vi "writeRequest.vi"(5 "id":u16, 7 "cmd":string, 9 "data":string) -> (8 "readRequest":string)   [LabVIEW 2015, in "labOpenShowVar.lvlib"]
uses:
  labOpenShowVar.lvlib
panel:
  out "输出":u8[](array[numeric]) format="%02d"
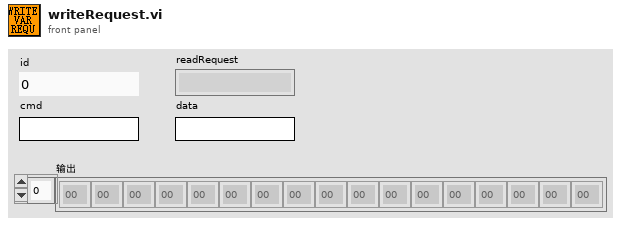
[diagram p1: front panel]
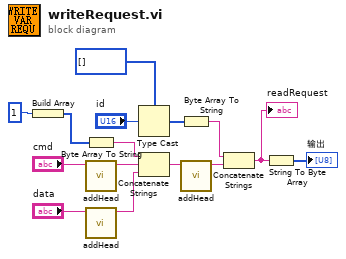
[diagram p0: block diagram]
diagram:
  n1 = Build Array(u8 1) -> (w9:u8[])
  n2 = Byte Array To String(unsigned byte array=w9) -> (string=w12:string)
  n3 = call "addHead.vi"("cmd"="cmd") -> ("添加后"=w13:string)  [unwired: 10 in]
  n4 = call "addHead.vi"("cmd"="data") -> ("添加后"=w1:string)  [unwired: 10 in]
  n5 = Type Cast(type=u8[] [], x="id") -> (*(type *) &x=w3:u8[])
  n6 = Concatenate Strings(w12, w13, w1) -> (w11:string)
  n7 = Byte Array To String(unsigned byte array=w3) -> (string=w6:string)
  n8 = call "addHead.vi"("cmd"=w11) -> ("添加后"=w8:string)  [unwired: 10 in]
  n9 = Concatenate Strings(w6, w8) -> (w7:string)
  "readRequest" <- w7
  n10 = String To Byte Array(string=w7) -> (unsigned byte array=→"输出":u8[])
